vi "Password Dialog.vi"(0 "Enable":bool=TRUE, 1 "IP Placeholder":string caption="IP address", 5 "error in (no error)":errorcluster) -> (15 "Password":string, 16 "Username":string, 17 "IP address":string, 18 "OK":bool, 19 "error out":errorcluster)   [LabVIEW 2017]
doc: "Displays a standard dialog box that prompts users to enter information, such as a user name and password.\n--------------------\n\nThis Express VI is configured as follows:\n\nMessage to Display to the User:RIO File Transfer Credentials\nThe inputs are: \nText Entry Box: IP address\nText Entry Box: Username\nText Entry Box: Password"
panel:
  in  "Password":string
  in  "Username":string
  in  "IP address":string
  out "String":string="RIO File Transfer Credentials"
  in  "Cancel":bool
  in  "OK2":bool
  in  "OK1":bool
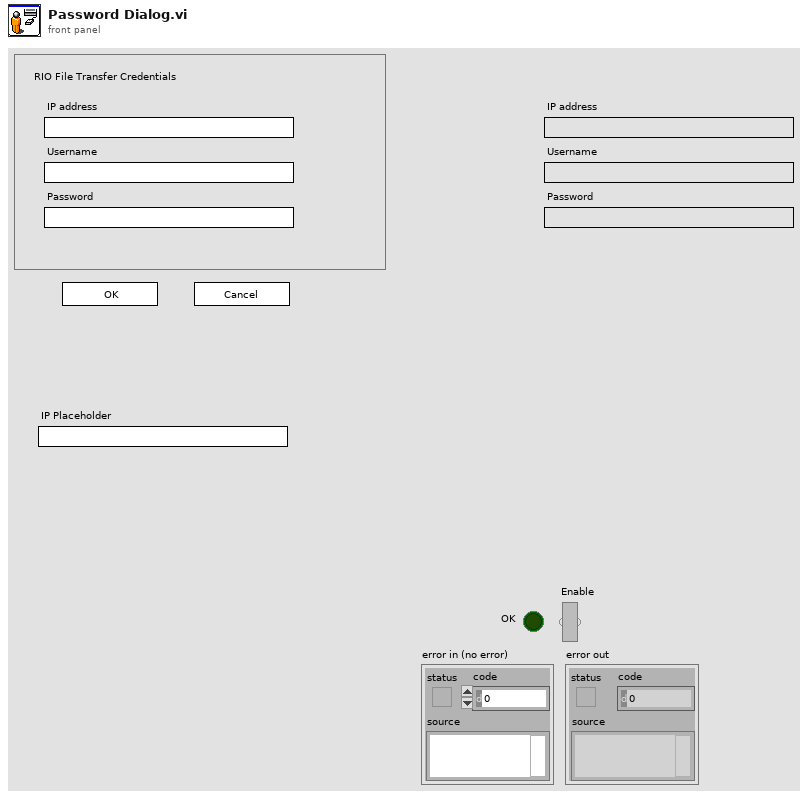
[diagram p1: front panel]
types:
  T1 = cluster{"Input Name":string, "Input Data Type":i32}[]
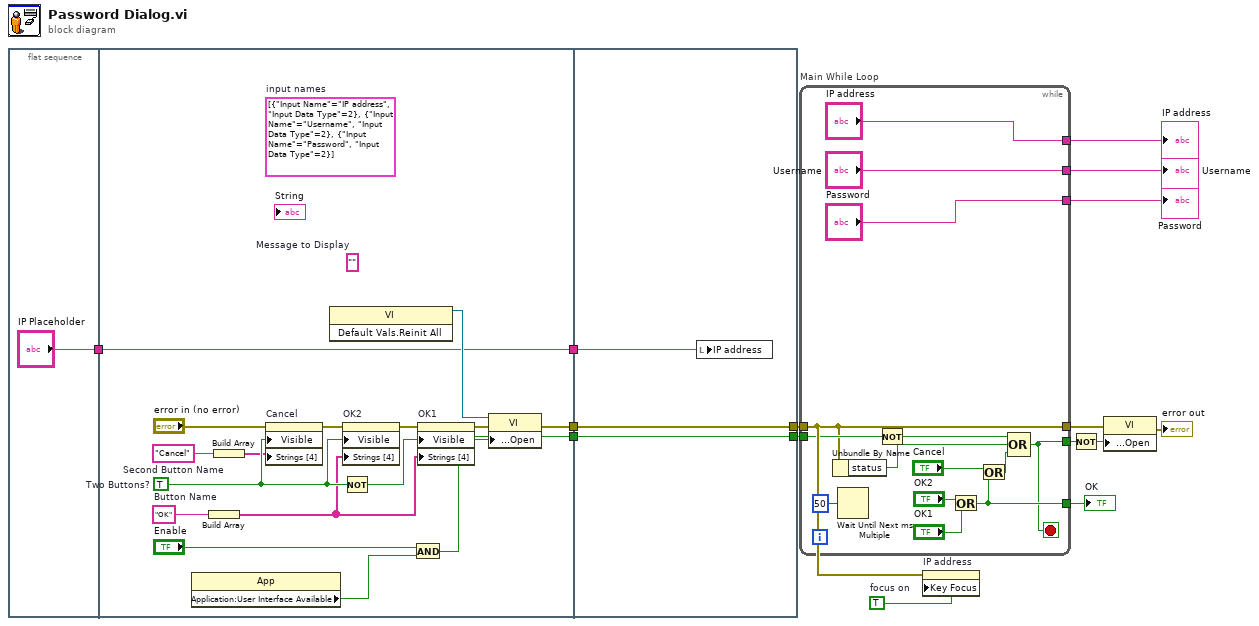
[diagram p0: block diagram]
diagram:
  w7 = TRUE  # focus on
  n1 = flat-sequence {
    tunnel: ["IP Placeholder"] -> w1
    tunnel: [w23] -> w4
    tunnel: [w20] -> w3
    tunnel: [w17] -> w2
    tunnel: w1 -> [w17]
    tunnel: [w34] -> w9
    tunnel: [w35] -> w12
    tunnel: w4 -> [w35]
    tunnel: w3 -> [w34]
    tunnel: w2 -> [w33]
    frame #0 {
    }
    frame #1 {
      (unwired) T1 [{"Input Name"="IP address", "Input Data Type"=2}, {"Input Name"="Username", "Input Data Type"=2}, {"Input Name"="Password", "Input Data Type"=2}]  # input names
      w27 = "Cancel"  # Second Button Name
      w25 = "OK"  # Button Name
      (unwired) ""  # Message to Display
      w32 = TRUE  # Two Buttons?
      n2 = property class="App"() -> ("Application:User Interface Available"=w19:bool)  [unwired: 2 in, 2 out]
      n3 = Build Array(w25) -> (w26:string[])
      n4 = Build Array(w27) -> (w28:string[])
      n5 = property on="Cancel" class="Bool"(error in="error in (no error)", "Visible"=w32, "Strings [4]"=w28) -> (error out=w30:errorcluster)  [unwired: 1 in, 1 out]
      n6 = invoke class="VI" method="Default Vals.Reinit All"() -> (reference out=w18:refnum<vi>)  [unwired: 3 in, 2 out]
      n7 = Not(x=w32) -> (.not. x?=w31:bool)
      n8 = property on="OK2" class="Bool"(error in=w30, "Visible"=w32, "Strings [4]"=w26) -> (error out=w29:errorcluster)  [unwired: 1 in, 1 out]
      n9 = And(x="Enable", y=w19) -> (x .and. y?=w20:bool)
      n10 = property on="OK1" class="Bool"(error in=w29, "Visible"=w31, "Strings [4]"=w26) -> (error out=w24:errorcluster)  [unwired: 1 in, 1 out]
      n11 = property class="VI"(reference=w18, error in=w24, "Front Panel Window:Open"=w20) -> (error out=w23:errorcluster)  [unwired: 1 out]
    }
    frame #2 {
      n12 = local write "IP address"(w33) -> ()
    }
  }
  n13 = while "Main While Loop" {
    tunnel: [w46] -> w15
    tunnel: w9 -> [w44]
    tunnel: [w42] -> w13
    tunnel: w12 -> [w41]
    tunnel: [w41] -> w11
    tunnel: ["IP address"] -> w8
    tunnel: ["Username"] -> w6
    tunnel: ["Password"] -> w5
    stop <- w42 stop-if-true
    n14 = Unbundle By Name(w41) -> ("status"=w39:bool)
    n15 = Wait Until Next ms Multiple(millisecond multiple=u32 50) -> ()  [unwired: 1 out]
    n16 = Not(x=w44) -> (.not. x?=w43:bool)
    n17 = Or(x="OK2", y="OK1") -> (x .or. y?=w46:bool)
    n18 = Or(x="Cancel", y=w46) -> (x .or. y?=w40:bool)
    n19 = Compound Arithmetic op=OR(w43, w39, w40) -> (w42:bool)
  }
  "OK" <- w15
  "IP address" <- w8
  "Username" <- w6
  "Password" <- w5
  n20 = property on="IP address" class="Str"(error in=w12, "Key Focus"=w7) -> ()  [unwired: 1 in, 2 out]
  n21 = Not(x=w13) -> (.not. x?=w14:bool)
  n22 = property class="VI"(error in=w11, "Front Panel Window:Open"=w14) -> (error out=→"error out":errorcluster)  [unwired: 1 in, 1 out]
